vi "GDS_MO_SetEnergy170622.vi"(11 "AEnergy":dbl=8.0) -> ()   [LabVIEW 2015]
uses:
  C/Program Files/National Instruments/LabVIEW 2015/user.lib/caLab/Private/Get_PV-1D.vi
  C/Program Files/National Instruments/LabVIEW 2015/user.lib/caLab/Private/Put_DBL-1D_PV-1D.vi
  C/Program Files/National Instruments/LabVIEW 2015/user.lib/caLab/Private/Put_DBL_PV.vi
  C/Program Files/National Instruments/LabVIEW 2015/user.lib/caLab/Private/Get_PV.vi
panel:
  out "1rst Value (number) 2":dbl
  out "1rst Value (number)":dbl
  out "SPEC:BUSY":dbl
  out "SPEC:INC":dbl
  out "retrun value":i32
  out "SPEC:ExpNumber_RV":dbl=99.0
  # "SetEnergy"
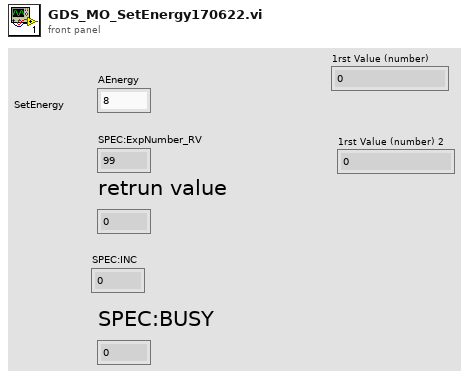
[diagram p1: front panel]
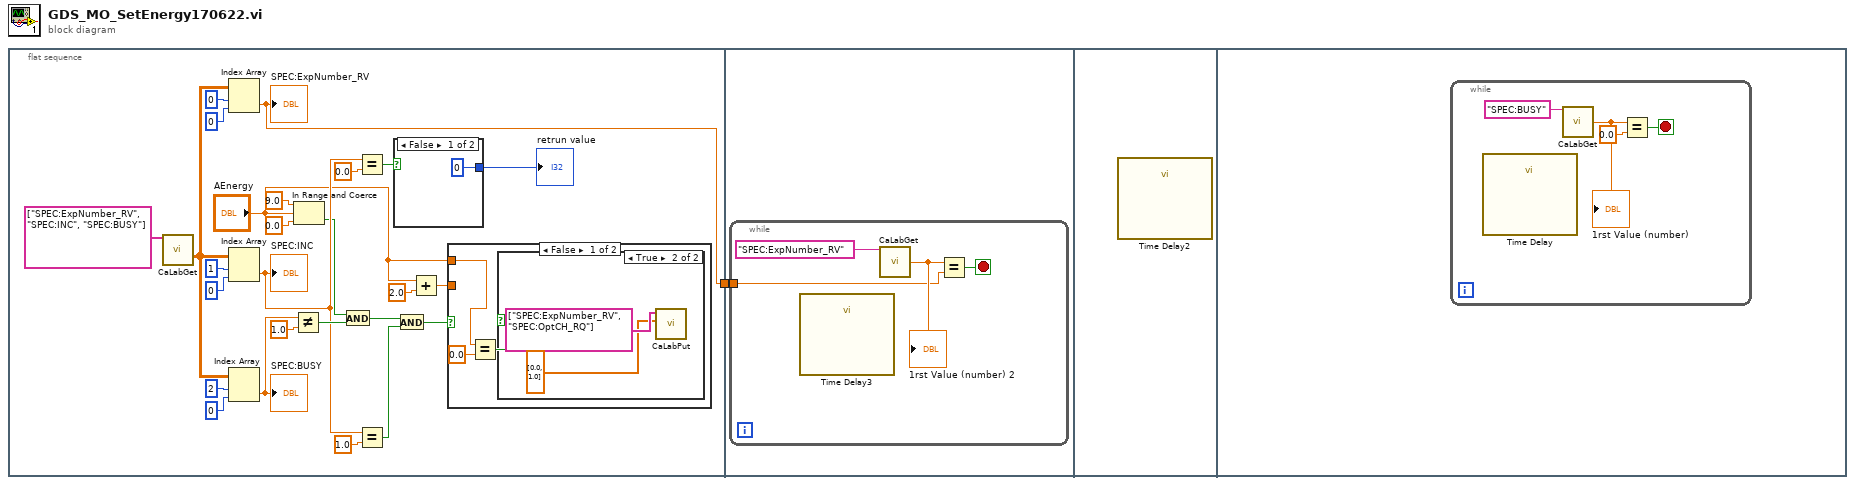
[diagram p0: block diagram]
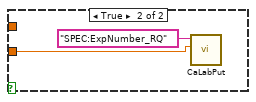
[diagram p3: hidden frame]
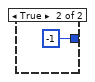
[diagram p4: hidden frame]
diagram:
  n1 = flat-sequence {
    tunnel: [w3] -> w1
    tunnel: w1 -> [w37]
    frame #0 {
      n2 = call-poly "CaLabGet.vi"("PV Names"=string[] ["SPEC:ExpNumber_RV", "SPEC:INC", "SPEC:BUSY"]) -> ("Value Array (number)"=w20:dbl[][])  [unwired: 8 in, 6 out]
      n3 = Index Array(array=w20, index (row)=0, index (col)=0 ("disabled index (col)")) -> (element=w3:dbl)
      "SPEC:ExpNumber_RV" <- w3
      n4 = Index Array(array=w20, index (row)=1, index (col)=0 ("disabled index (col)")) -> (element=w14:dbl)
      "SPEC:INC" <- w14
      n5 = Index Array(array=w20, index (row)=2, index (col)=0 ("disabled index (col)")) -> (element=w4:dbl)
      "SPEC:BUSY" <- w4
      n6 = Not Equal?(x=w4, y=1.0) -> (x != y?=w15:bool)
      n7 = In Range and Coerce(upper limit=9.0, x="AEnergy", lower limit=0.0) -> (In Range?=w5:bool)  [unwired: 1 out]
      n8 = And(x=w5, y=w15) -> (x .and. y?=w12:bool)
      n9 = Equal?(x=w14, y=0.0) -> (x = y?=w18:bool)
      n10 = Equal?(x=w14, y=1.0) -> (x = y?=w11:bool)
      n11 = case shown="False" w18 {
        tunnel: [0 -1] -> w17
        frame False {
        }
        frame True {
        }
      }
      "retrun value" <- w17
      n12 = And(x=w12, y=w11) -> (x .and. y?=w10:bool)
      n13 = Add(x="AEnergy", y=2.0) -> (x+y=w8:dbl)
      n14 = case shown="False" w10 {
        tunnel: w8 -> [_ w33]
        tunnel: "AEnergy" -> [w28 _]
        frame False {
          n15 = Equal?(x=w28, y=0.0) -> (x = y?=w30:bool)
          n16 = case shown="True" w30 {
            frame False {
            }
            frame True {
              n17 = call-poly "CaLabPut.vi"("Values"=dbl[] [0.0, 1.0] ("PV Names"), "PV Names"=string[] ["SPEC:ExpNumber_RV", "SPEC:OptCH_RQ"]) -> ()  [unwired: 6 in, 4 out]
            }
          }
        }
        frame True {
          n18 = call-poly "CaLabPut.vi"("Value"=w33, "PV Name"="SPEC:ExpNumber_RQ") -> ()  [unwired: 6 in, 4 out]
        }
      }
    }
    frame #1 {
      n19 = while {
        tunnel: w37 -> [w38]
        stop <- w41 stop-if-true
        n20 = call "Time Delay3"() -> ()  [unwired: 11 in, 1 out]
        n21 = call-poly "CaLabGet.vi"("PV Name"="SPEC:ExpNumber_RV") -> ("1rst Value (number)"=w39:dbl)  [unwired: 8 in, 6 out]
        "1rst Value (number) 2" <- w39
        n22 = Equal?(x=w39, y=w38) -> (x = y?=w41:bool)
      }
    }
    frame #2 {
      n23 = call "Time Delay2"() -> ()  [unwired: 11 in, 1 out]
    }
    frame #3 {
      n24 = while {
        stop <- w45 stop-if-true
        n25 = call "Time Delay"() -> ()  [unwired: 11 in, 1 out]
        n26 = call-poly "CaLabGet.vi"("PV Name"="SPEC:BUSY") -> ("1rst Value (number)"=w42:dbl)  [unwired: 8 in, 6 out]
        "1rst Value (number)" <- w42
        n27 = Equal?(x=w42, y=0.0) -> (x = y?=w45:bool)
      }
    }
  }
